vi "action.vi"(0 "HGF_FGV_SelectByName":refnum<class "HGF_FGV_SelectByName.lvclass">, 2 "Objects":refnum<class>[](array[class]), 5 "error in (no error)":errorcluster) -> (14 "dup HGF_FGV_SelectByName":refnum<class "HGF_FGV_SelectByName.lvclass">, 16 "dup Objects":refnum<class>[](array[class]), 19 "error out":errorcluster)   [LabVIEW 2012, in "HGF_FGV.lvlib" / "HGF_FGV_SelectByName.lvclass"]
doc: "Return copy of selected objects from object array."
uses:
  HGF_FGV_SelectByName.lvclass
  HGF_Base/HGF_Base.lvclass
  HGF_FGV_SelectByName.lvclass/HGF_FGV_SelectByName.ctl
  HGF_Factory/HGF_Factory.lvclass
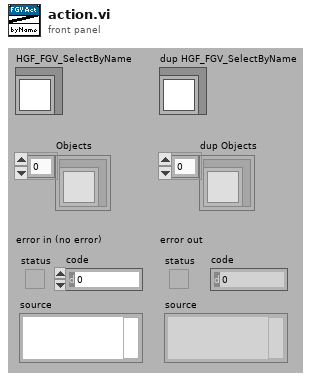
[diagram p1: front panel]
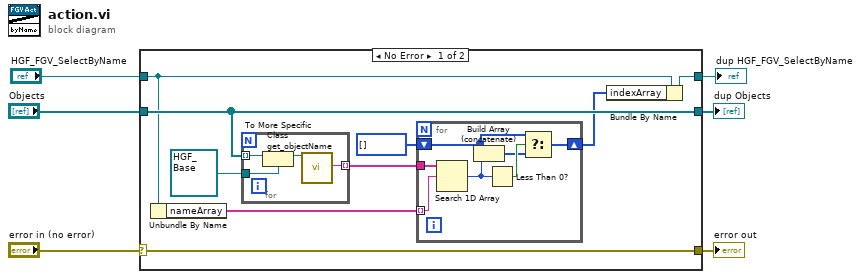
[diagram p0: block diagram]
diagram:
  n1 = case shown="No Error" "error in (no error)" {
    selector: "error in (no error)" -> [w10 w29]
    tunnel: [w10 w29] -> w5
    tunnel: [w8 w28] -> w3
    tunnel: "HGF_FGV_SelectByName" -> [w9 w28]
    tunnel: [w11 w27] -> w2
    tunnel: "Objects" -> [w11 w27]
    frame No Error {
      n2 = Unbundle By Name(w9) -> ("nameArray"=w14:string[])
      n3 = for {
        tunnel: w11 -> [w25] mode=indexing
        tunnel: refnum<class "HGF_Base.lvclass"> refnum ("HGF_BaseClasses.lvlib:HGF_Base.lvclass") -> [w24]
        tunnel: [w23] -> w13 mode=indexing
        n4 = To More Specific Class(target class=w24, reference=w25) -> (specific class reference=w26:refnum<class "HGF_Base.lvclass">)  [unwired: 1 in, 1 out]
        n5 = call "get_objectName.vi"("HGF_Factory"=w26) -> ("objectName"=w23:string)  [unwired: 1 in, 17 out]
      }
      n6 = for {
        tunnel: w14 -> [w21] mode=indexing
        tunnel: w13 -> [w22]
        shift-right: [w16] -> w7
        shift-left: u32[] [] -> [w19]
        n7 = Search 1D Array(1D array=w22, element=w21) -> (index of element=w17:i32)  [unwired: 1 out]
        n8 = Build Array (concatenate)(w19, w17) -> (w18:u32[])
        n9 = Less Than 0?(x=w17) -> (x < 0?=w20:bool)
        n10 = Select(t=w19, s=w20, f=w18) -> (s? t:f=w16:u32[])
      }
      n11 = Bundle By Name(cluster=w9, "indexArray"=w7) -> (w8:refnum<class "HGF_FGV_SelectByName.lvclass">)
    }
    frame Error {
    }
  }
  "error out" <- w5
  "dup HGF_FGV_SelectByName" <- w3
  "dup Objects" <- w2
